vi "Rosliny_zmienne.vi"() -> ()   [LabVIEW 2023]
panel:
  in  "Ustaw czas podlewania harmonogram":dbl
  in  "Czas podlewania harmonogram":dbl
  in  "Czas podlewania reczny":dbl
  in  "Ustaw":bool
  in  "Ustaw czas podlewania reczny":dbl
  in  "Podlewaj tryb reczny":bool
  in  "Podlewaj":bool
  in  "Liczba sekcji":dbl
  in  "Minuta":i32=4
  in  "Godzina":i32=1
  in  "Rok":dbl
  in  "Miesiac":dbl
  in  "Dzien":dbl
  in  "Czas podlewania":dbl
  in  "Powierzchnia":dbl
  in  "Ilosc zraszaczy":dbl
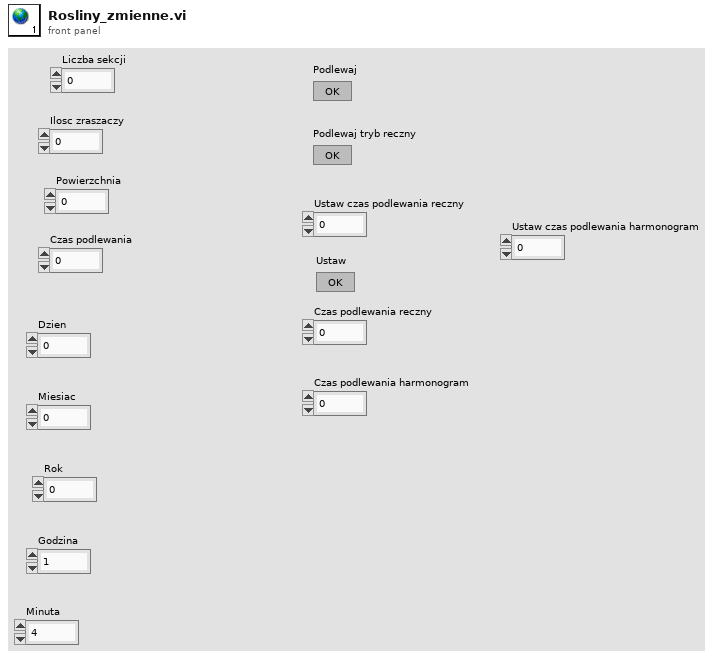
[diagram p1: front panel]
diagram:
